vi "Zmag to F.vi"(9 "Z 输入":dbl, 11 "Parameter T1":cluster{"A":dbl, "B":dbl}={"A"=28.06, "B"=-1.501}) -> (2 "F 输出":dbl)   [LabVIEW 2017]
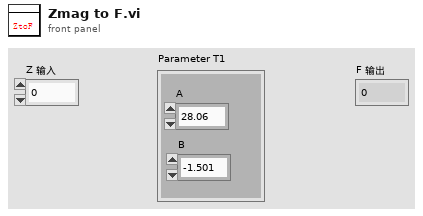
[diagram p1: front panel]
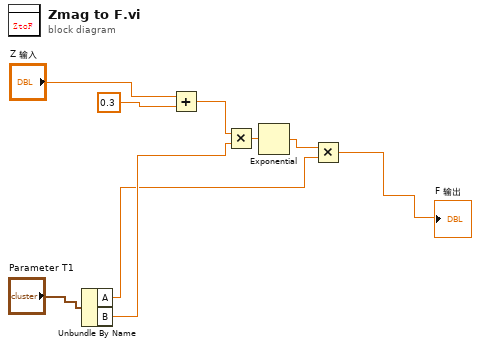
[diagram p0: block diagram]
diagram:
  n1 = Unbundle By Name("Parameter T1") -> ("A"=w5:dbl, "B"=w6:dbl)
  n2 = Add(x="Z 输入", y=0.3) -> (x+y=w1:dbl)
  n3 = Multiply(x=w1, y=w6) -> (x*y=w8:dbl)
  n4 = Exponential(1:w8) -> (0:w9:dbl)
  n5 = Multiply(x=w9, y=w5) -> (x*y=→"F 输出":dbl)
